vi "ResizeGraphtoPane.vi"(4 "Force aspect ratio?":bool, 5 "Borders in Percent(T) or Pixels (F)":bool, 6 "Adjust":u16(ring) items=["Height", "Width", "Both"], 7 "Minimal":T1, 8 "error in (no error)":errorcluster, 9 "Borders":T2, 10 "Graph Chart":refnum<vi>, 11 "PentaPanesGUI in":refnum<class "PentaPanes.lvclass">) -> (0 "error out":errorcluster, 3 "PentaPanesGUI out":refnum<class "PentaPanes.lvclass">)   [LabVIEW 2022 SP3, in "PentaPanesLibrary.lvlib" / "PentaPanes.lvclass"]
uses:
  PentaPanes.lvclass
  BordersCluster.ctl
  <vilib>/Utility/miscctls.llb/LVBoundsTypeDef.ctl
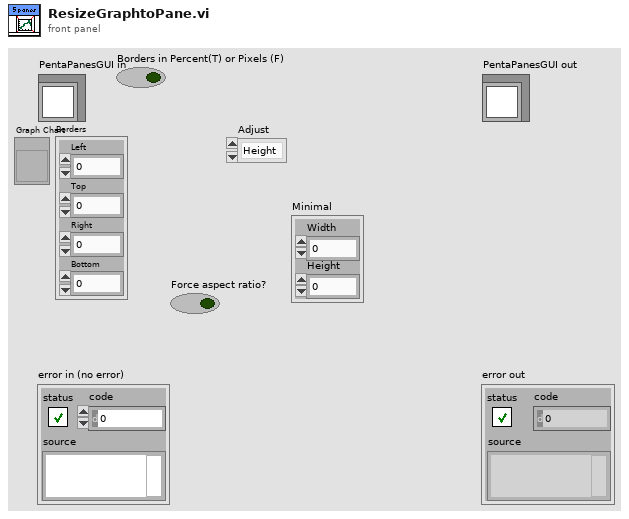
[diagram p1: front panel]
types:
  T1 = typedef "LVBoundsTypeDef.ctl" = cluster{"Width":i32, "Height":i32}
  T2 = typedef "PentaPanesLibrary.lvlib/PentaPanes.lvclass/BordersCluster.ctl" = cluster{"Left":i32, "Top":i32, "Right":i32, "Bottom":i32}
  T3 = typedef "LVBoundsTypeDef.ctl" = cluster{"Width":u32, "Height":u32}
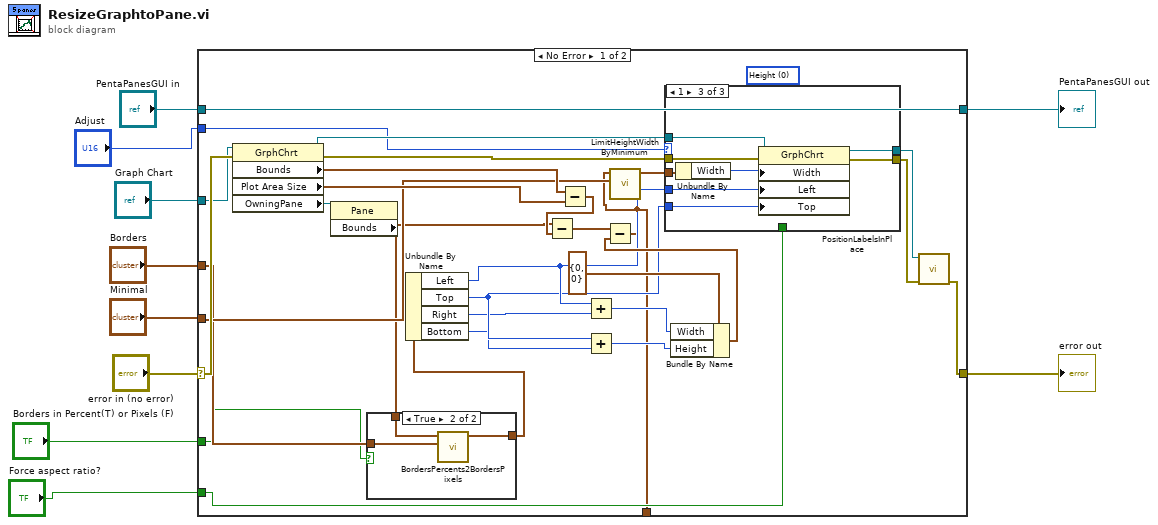
[diagram p0: block diagram]
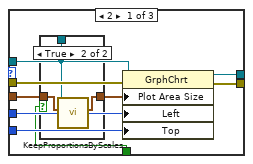
[diagram p3: hidden frame]
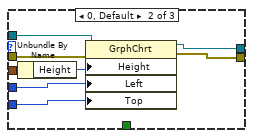
[diagram p5: hidden frame]
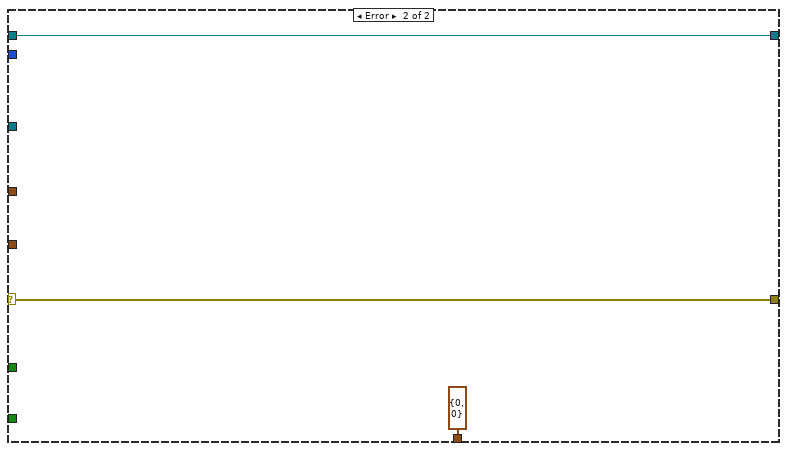
[diagram p6: hidden frame]
diagram:
  n1 = case shown="No Error" "error in (no error)" {
    selector: "error in (no error)" -> [w34 w76]
    tunnel: [w13 w76] -> w9
    tunnel: [w40 w75] -> w7
    tunnel: "PentaPanesGUI in" -> [w40 w75]
    tunnel: "Graph Chart" -> [w12 _]
    tunnel: "Borders" -> [w19 _]
    tunnel: "Adjust" -> [w27 _]
    tunnel: "Minimal" -> [w25 _]
    tunnel: "Borders in Percent(T) or Pixels (F)" -> [w17 _]
    tunnel: "Force aspect ratio?" -> [w16 _]
    tunnel: [w15 T1 {"Width"=0, "Height"=0} ("Bounds")] -> _
    frame No Error {
      (unwired) u16 0 items=["Height", "Width", "Both"] ("Adjust")
      n2 = property class="GrphChrt"(reference=w12, error in=w34) -> (reference out=w35:refnum<vi>, error out=w28:errorcluster, "Bounds"=w39:T3, "Plot Area Size"=w38:T3, "OwningPane"=w36:refnum<vi>)
      n3 = property class="Pane"(reference=w36) -> ("Bounds"=w22:T3)  [unwired: 1 in, 2 out]
      n4 = case shown="True" w17 {
        tunnel: w22 -> [_ w44]
        tunnel: w19 -> [w41 w43]
        tunnel: [w41 w42] -> w18
        frame False {
        }
        frame True {
          n5 = call "BordersPercents2BordersPixels.vi"("Borders in"=w43, "Bounds"=w44) -> ("Borders out"=w42:T2)  [unwired: 9 in]
        }
      }
      n6 = Unbundle By Name(w18) -> ("Left"=w24:i32, "Top"=w23:i32, "Right"=w21:i32, "Bottom"=w20:i32)
      n7 = Subtract(x=w39, y=w38) -> (x-y=w37:T3)
      n8 = Subtract(x=w22, y=w37) -> (x-y=w30:T3)
      n9 = Add(x=w24, y=w21) -> (x+y=w32:i32)
      n10 = Add(x=w23, y=w20) -> (x+y=w31:i32)
      n11 = Bundle By Name(cluster=T1 {"Width"=0, "Height"=0} ("x-y"), "Width"=w32, "Height"=w31) -> (w29:T1)
      n12 = Subtract(x=w30, y=w29) -> (x-y=w15:T3)
      n13 = call "LimitHeightWidthByMinimum.vi"("Minimal"=w25, "Height Width in"=w15) -> ("Limited Height Width out"=w26:T1)  [unwired: 9 in]
      n14 = case shown="1" w27 {
        tunnel: w35 -> [w46 w65 w73]
        tunnel: w26 -> [w49 w60 w68]
        tunnel: w24 -> [w53 w64 w72]
        tunnel: w23 -> [w52 w63 w71]
        tunnel: w28 -> [w51 w62 w70]
        tunnel: [w50 w61 w69] -> w14
        tunnel: w16 -> [w47 _ _]
        tunnel: [w45 w58 w66] -> w11
        frame 2 {
          n15 = case shown="True" w47 {
            tunnel: w49 -> [w54 w57]
            tunnel: [w54 w56] -> w48
            tunnel: w46 -> [_ w55]
            frame False {
            }
            frame True {
              n16 = call "KeepProportionsByScales.vi"("Bounds in"=w57, "GraphChart in"=w55) -> ("Bounds out"=w56:T1)  [unwired: 5 in, 4 out]
            }
          }
          n17 = property class="GrphChrt"(reference=w46, error in=w51, "Plot Area Size"=w48, "Left"=w53, "Top"=w52) -> (reference out=w45:refnum<vi>, error out=w50:errorcluster)
        }
        frame 0, Default {
          n18 = Unbundle By Name(w60) -> ("Height"=w59:i32)
          n19 = property class="GrphChrt"(reference=w65, error in=w62, "Height"=w59, "Left"=w64, "Top"=w63) -> (reference out=w58:refnum<vi>, error out=w61:errorcluster)
        }
        frame 1 {
          n20 = Unbundle By Name(w68) -> ("Width"=w67:i32)
          n21 = property class="GrphChrt"(reference=w73, error in=w70, "Width"=w67, "Left"=w72, "Top"=w71) -> (reference out=w66:refnum<vi>, error out=w69:errorcluster)
        }
      }
      n22 = call "PositionLabelsInPlace.vi"("error in (no error)"=w14, "XYGraph in"=w11) -> ("error out"=w13:errorcluster)  [unwired: 9 in]
    }
    frame Error {
    }
  }
  "error out" <- w9
  "PentaPanesGUI out" <- w7
